vi "Entre_24_0.vi"(6 "Min":dbl, 7 "Max":dbl=24.0, 11 "Entrée":dbl) -> (3 "Sortie":dbl)   [LabVIEW 2019]
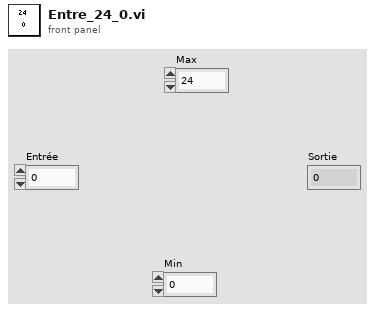
[diagram p1: front panel]
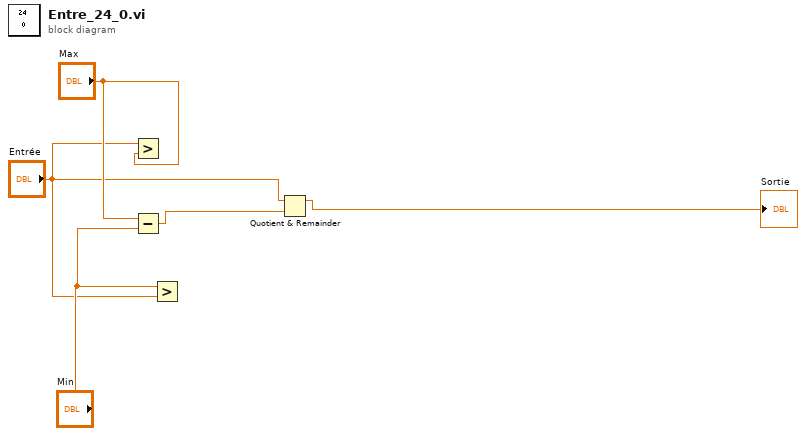
[diagram p0: block diagram]
diagram:
  n1 = Greater?(x="Entrée", y="Max") -> ()  [unwired: 1 out]
  n2 = Subtract(x="Max", y="Min") -> (x-y=w2:dbl)
  n3 = Greater?(x="Min", y="Entrée") -> ()  [unwired: 1 out]
  n4 = Quotient & Remainder(x="Entrée", y=w2) -> (x-y*floor(x/y)=→"Sortie":dbl)  [unwired: 1 out]
